vi "RSNRPZ Configure Timeslot.vi"(7 "Width (1.0e-3 s)":dbl=0.001 format="%.2p", 8 "error in (no error)":errorcluster, 9 "Time Slot Count (8)":i32=8, 10 "Channel (1)":i32=1, 11 "VISA session":refnum<visa-resource-name> caption="VISA resource name") -> (0 "error out":errorcluster, 3 "dup VISA session":refnum<visa-resource-name> caption="VISA resource name")   [LabVIEW 2010]
doc: "This VI configures the parameters of Timeslot measurement mode. Both exclude start and stop are set to 10% of timeslot width each.\n\nRemote-control command(s):\nSENS:POW:TSL:AVG:COUN\nSENS:POW:TSL:AVG:WIDT\nSENS:TIM:EXCL:STAR\nSENS:TIM:EXCL:STOP"
uses:
  rsnrpz_32.dll
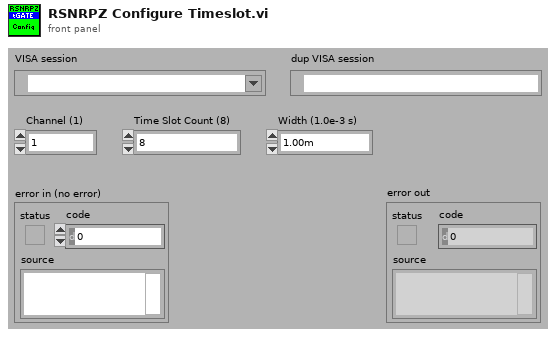
[diagram p1: front panel]
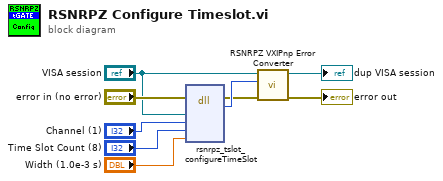
[diagram p0: block diagram]
diagram:
  n1 = dll-call lib="rsnrpz_32.dll" fn="rsnrpz_tslot_configureTimeSlot"(error in="error in (no error)", "VISA Session"="VISA session", "Channel"="Channel (1)", "Time Slot Count"="Time Slot Count (8)", "Width"="Width (1.0e-3 s)") -> (error out=w5:errorcluster, "Status"=w9:i32)  [unwired: 6 in, 1 out]
  n2 = call <instrlib>:"RSNRPZ VXIPnp Error Converter.vi"("error in"=w5, "VXIPnp error code"=w9, "VISA session"="VISA session") -> ("error out"=→"error out":errorcluster, "dup VISA session"=→"dup VISA session":refnum<visa-resource-name>)  [unwired: 7 in]
